vi "Range Destroy.vi"(8 "error in (no error)":errorcluster, 11 "Range DVR in":refnum<data-value>) -> (0 "error out":errorcluster)   [LabVIEW 2010, in "MDSplus.lvlib"]
uses:
  <vilib>/MDSplus/Library/MDSplus.lvlib
  <vilib>/MDSplus/Classes/Data_Class/Compound_Class/Range_Class/Range.lvclass
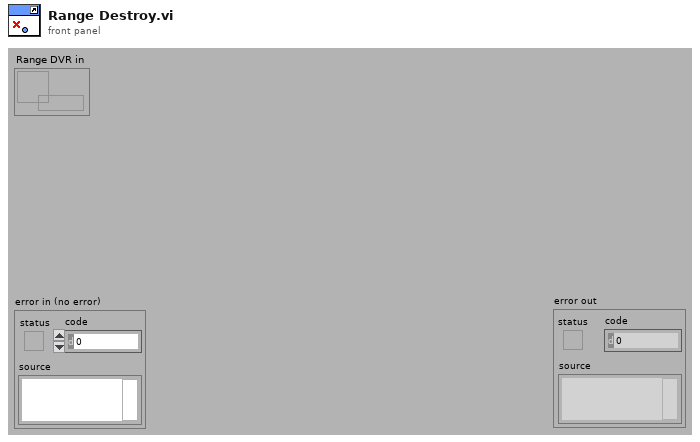
[diagram p1: front panel]
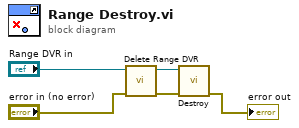
[diagram p0: block diagram]
diagram:
  n1 = call <vilib>:"Delete Range DVR.vi"("error in (no error)"="error in (no error)", "Range DVR in"="Range DVR in") -> ("error out"=w3:errorcluster, "Range out"=w1:refnum<class "Range.lvclass">)  [unwired: 8 in]
  n2 = call-dynamic "Destroy.vi"("error in (no error)"=w3, "Range in"=w1) -> ("error out"=→"error out":errorcluster)  [unwired: 9 in]
